vi "Motion_Convert Register to Int.vi"(5 "Register array":u16[](array[numeric])) -> (6 "Int":u32)   [LabVIEW 2010]
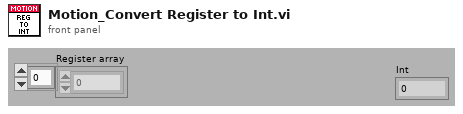
[diagram p1: front panel]
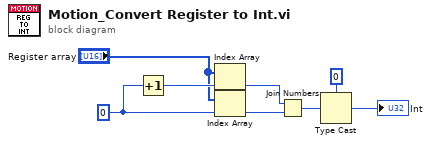
[diagram p0: block diagram]
diagram:
  w3 = 0 ("Start index")
  n1 = Increment(x=w3) -> (x+1=w4:i32)
  n2 = Index Array(array="Register array", index=w4) -> (element=w8:u16)
  n3 = Index Array(array="Register array", index=w3) -> (element=w7:u16)
  n4 = Join Numbers(hi=w8, lo=w7) -> ((hi.lo)=w1:u32)
  n5 = Type Cast(type=u32 0, x=w1) -> (*(type *) &x=→"Int":u32)
